vi "Create.vi"(8 "error in (no error)":errorcluster) -> (0 "error out":errorcluster, 3 "Ignore Inputs Comparator":refnum<class "Any Inputs Comparator.lvclass">)   [LabVIEW 2020, in "Any Inputs Comparator.lvclass"]
uses:
  Any Inputs Comparator.lvclass
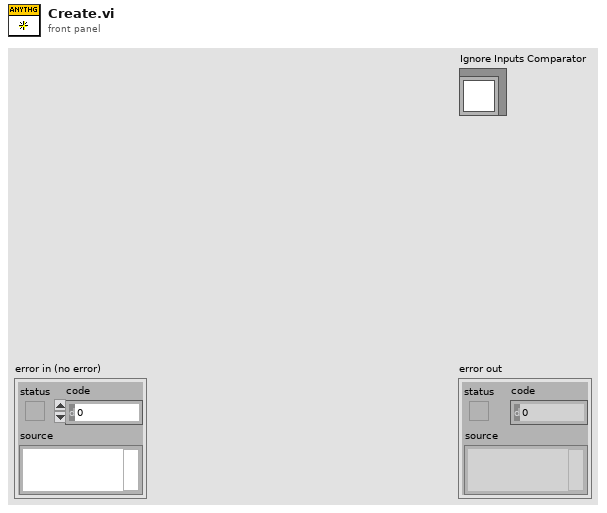
[diagram p1: front panel]
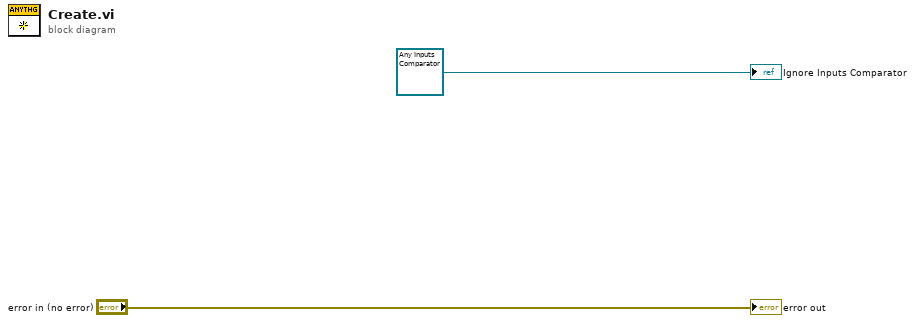
[diagram p0: block diagram]
diagram:
  "error out" <- "error in (no error)"
  "Ignore Inputs Comparator" <- refnum<class "Any Inputs Comparator.lvclass"> refnum ("Ignore Inputs Comparator")
